vi "Chroma 1905x Series Preset Lot Number.vi"(2 "error in":T1, 3 "Lot Number":string, 4 "inst handle in":refnum<visa-resource-name>) -> (0 "error out":T1, 1 "inst handle out":refnum<visa-resource-name>)   [LabVIEW 2025]
doc: "Contact Chroma\nTEL: +886-2-2298-3855 \nTEL: +886-3-397-5788 \nFAX: +886-2-2298-3596\nFAX: +886-3-327-4703 \nURL: http://www.chromaate.com \nE-mail: chroma@chroma.com.tw"
uses:
  <instrlib>/Chroma 19052/Chroma 19052.lvlib
panel:
  # "Lot Number\nNo More than 9 Characters"
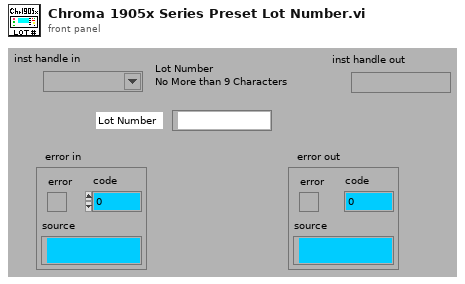
[diagram p1: front panel]
types:
  T1 = cluster{"error":bool, "code":i8, "source":string}
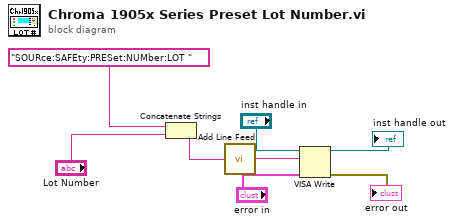
[diagram p0: block diagram]
diagram:
  n1 = Concatenate Strings("SOURce:SAFEty:PRESet:NUMber:LOT ", "Lot Number") -> (w2:string)
  n2 = call <instrlib>:"Add Line Feed.vi"("Cmdstring"=w2) -> ("Concatenated String"=w1:string)
  n3 = VISA Write(VISA resource name="inst handle in", write buffer=w1, error in (no error)="error in") -> (VISA resource name out=→"inst handle out":refnum<visa-resource-name>, error out=→"error out":errorcluster)  [unwired: 1 out]
